vi "Factory Create.vi"(8 "Error In":errorcluster, 10 "IConfigure":refnum<class "IConfigure.lvclass">, 11 "reference in":refnum<class "FGen Simulated.lvclass">) -> (0 "Error Out":errorcluster, 3 "reference out":refnum<class "FGen Simulated.lvclass">)   [LabVIEW 2023, in "FGen Simulated.lvlib" / "FGen Simulated.lvclass"]
uses:
  FGen Simulated.lvclass
  FGen Simulated.lvclass/FGen Simulated.ctl
  Interfaces/IConfigure/IConfigure.lvclass
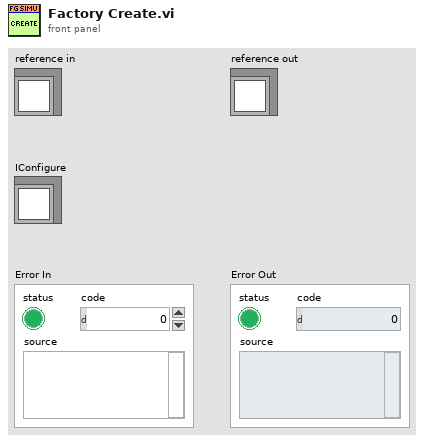
[diagram p1: front panel]
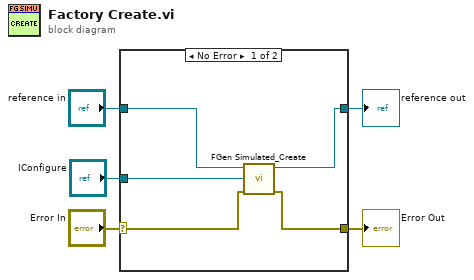
[diagram p0: block diagram]
diagram:
  n1 = case shown="No Error" "Error In" {
    selector: "Error In" -> [w6 w12]
    tunnel: [w7 w12] -> w4
    tunnel: [w8 w11] -> w2
    tunnel: "reference in" -> [w9 w11]
    tunnel: "IConfigure" -> [w10 _]
    frame No Error {
      n2 = call "FGen Simulated_Create.vi"("Error In"=w6, "IConfigure.lvclass"=w10, "reference in"=w9) -> ("Error Out"=w7:errorcluster, "reference out"=w8:refnum<class "FGen Simulated.lvclass">)  [unwired: 7 in]
    }
    frame Error {
    }
  }
  "Error Out" <- w4
  "reference out" <- w2
